vi "Append Image.vi"(0 "PDF Report IN":T24(xcontrol), 1 "Scale (%)":sgl=100.0, 3 "Border":T3={"Show?"=FALSE, "Thickness (point)"=0.5, "Color"=0}, 5 "Image path":path, 9 "Image Ref iTexSharp":refnum<k24>, 11 "error in (no error)":errorcluster, 12 "Caption":string, 14 "Position and indentation":T1={"Alignment"=enum."Center", "X "=0.0, "Y"=0.0, "Indentation"=0.0}) -> (4 "PDF Report OUT":T24(xcontrol), 6 "Image path duplicate":path, 8 "Size (points)":cluster{"TotalHeight":sgl, "TotalWidth":sgl}, 15 "error out":errorcluster)   [LabVIEW 2012]
doc: "The <B>VI</B> appends, to the PDF report, the image from a file. \n\nValid formats: GIF, JPEG, PNG and BMP.\n\n<B>FRANÇAIS</B>\nLe <B>VI</B> ajoute, au rapport PDF, l'image provenant d'un fichier.\n\nFormats valides : GIF, JPEG, PNG et BMP.\n\nVersion 1.0\nDeveloped by Jean-Marc Simard\nCopyright © 2010, Exaprom Inc.\nAll rights reserved.\nLicense: BSD\n\nWith iTextSharp 4.1.6 (http://itextsharp.sourceforge.net)\nunder Mozilla Public License Version 1.1\n(http://www.mozilla.org/MPL/MPL-1.1.html)"
uses:
  C:/Users/MaxCorp/Documents/GitHub/TopView/DLL/itextsharp.dll
  GitHub/TopView/DLL/itextsharp.dll
  Controls/Font size.ctl
  Controls/Font color.ctl
  Controls/Font cluster.ctl
  Controls/Texte alignement.ctl
  Controls/Line spacing.ctl
  Controls/Paragraphe cluster.ctl
  Controls/Image aligment.ctl
  Controls/Image border.ctl
  Controls/PDF Report Xcontrol/PDF Report.xctl
  Controls/Image alignment and position.ctl
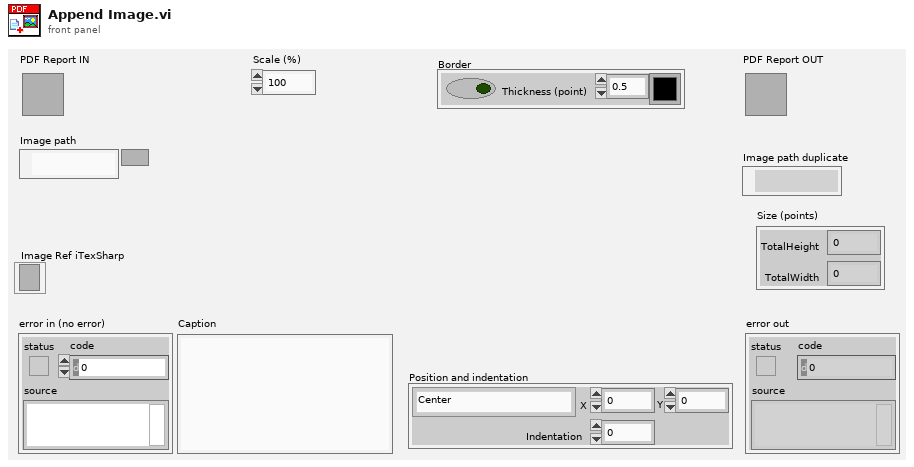
[diagram p1: front panel]
types:
  T1 = typedef "Image alignment and position.ctl" = cluster{"Alignment":T2, "X ":sgl, "Y":sgl, "Indentation":sgl}
  T2 = typedef "Image aligment.ctl" = enum16{"Absolute (X,Y) in mm", "Left", "Center", "Right", "Left (textwrap)", "Right (textwrap)"}
  T3 = typedef "Image border.ctl" = cluster{"Show?":bool, "Thickness (point)":sgl, "Color":u32}
  T4 = typedef "Font cluster.ctl" = cluster{"Name":string, "Size":T5, "Color":T6, "Style":cluster{"Bold":bool, "Italic":bool, "Underline":bool, "Strikeout":bool}}
  T5 = typedef "Font size.ctl" = sgl
  T6 = typedef "Font color.ctl" = u32
  T7 = typedef "Unit.ctl" = enum16{"inch", "mm"}
  T8 = typedef "Paragraphe cluster.ctl" = cluster{" Aligment":T9, "Line spacing":T10}
  T9 = typedef "Texte alignement.ctl" = enum16{"Select", "CENTER", "JUSTIFY", "LEFT", "RIGHT"}
  T10 = typedef "Line spacing.ctl" = enum16{"Select", "1.0", "1.5", "2.0"}
  T11 = typedef "Page dimensions.ctl" = cluster{"Start at page":i32, "Orientation":T12, "widht":sgl, "height":sgl, "Margin left":sgl, "Margin right":sgl, "Margin top":sgl, "Margin bottom":sgl}
  T12 = typedef "Page Orientation.ctl" = enum16{"Portrait", "Landscape"}
  T13 = typedef "Image or Table Caption.ctl" = cluster{"Caption":string, "Separator":string, "Position":enum16{"Above", "Below"}}
  T14 = typedef "Header Footer [ ].ctl" = T15[]
  T15 = typedef "Header Footer cluster.ctl" = cluster{"Start page":i32, "Type":T16, "Alignment":T17, "Vertical Alignement":T18, "Image (%)":sgl, "Page #":T19, "Text":string, "Path":string, "Font":T4, "Font refnum":refnum<k24>, "Line":cluster{"Line":T20, "Thickness (points)":sgl, "Colour":T6}}
  T16 = typedef "Header Footer Type.ctl" = enum16{"Select", "Text", "Text + hyperlink", "Page number", "Image", "Image + hyperlink"}
  T17 = typedef "Header footer horiz alignment.ctl" = enum16{"Left", "Center", "Right"}
  T18 = typedef "Cell Vertical alignment.ctl" = enum16{"TOP", "MIDDLE", "BOTTOM"}
  T19 = typedef "Page number.ctl" = cluster{"Text 1":string, "Text 2":string, "Text 3":string}
  T20 = typedef "Header Footer Line.ctl" = enum16{"No line", "Horizontal line"}
  T21 = typedef "Watermark cluster2.ctl" = cluster{"Show? (F)":bool, "Type":enum16{"Image", "Text"}, "Opacity (%)":sgl, "Rotate(°)":sgl, "Position":cluster{"Position":T22, "X":sgl, "Y":sgl}, "Image path":path, "Scaled(%)":sgl, "Image refnum":refnum<k24>, "Text":string, "Font":cluster{"Name":string, "Size":T5, "Color":T6}, "Font refnum":refnum<k24>, "Alignment":T17, "Automatic":bool}
  T22 = typedef "Watermark Position.ctl" = enum16{"Absolute", "Center (page)", "Center (text section)"}
  T23 = typedef "System Fonts.ctl" = cluster{"Font name [ ]":string[], "Font and file names [ ]":cluster{"Font name":string, "File name":string}[]}
  T24 = cluster{"Document":refnum<k24>, "Writer":refnum<k24>, "Default Font":refnum<k24>, "Default Font cluster":T4, "Path":path, "Unit (default = mm)":T7, "Paragraphe cluster":T8, "Pages dimensions [ ]":T11[], "Captions":cluster{"Image":T13, "Image counter":u16, "Table":T13, "Table counter":u16, "Font":T4}, "Header":T14, "Footer":T14, "Watermark ":T21, "Actual VI name":string, "System Fonts":T23}
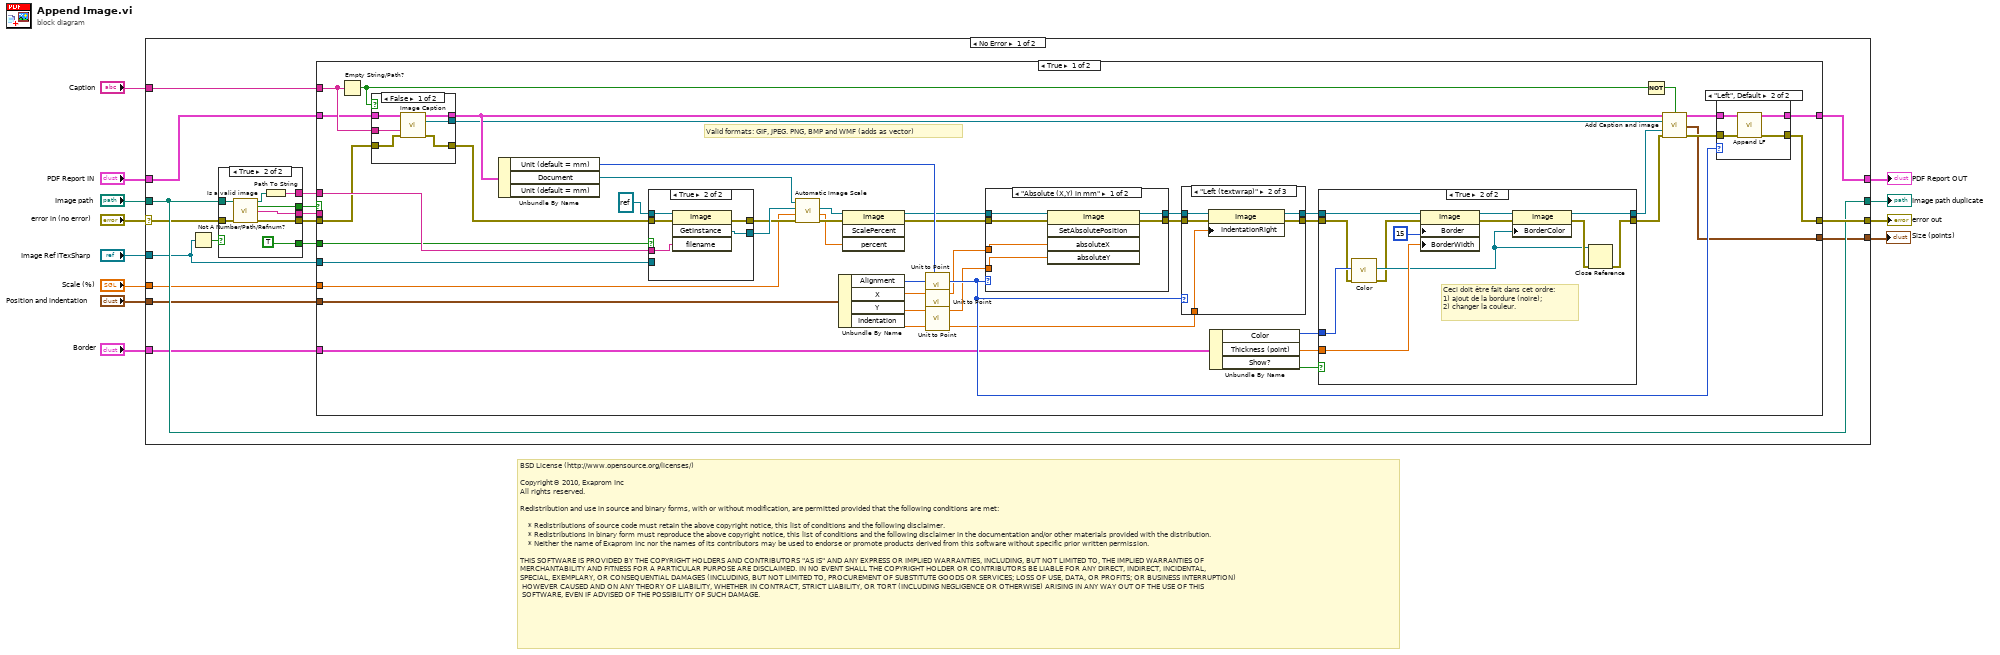
[diagram p0: block diagram]
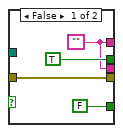
[diagram p2: hidden frame]
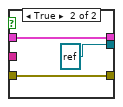
[diagram p5: hidden frame]
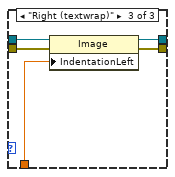
[diagram p7: hidden frame]
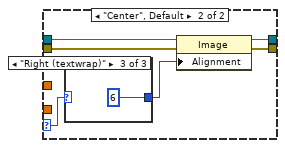
[diagram p9: hidden frame]
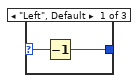
[diagram p10: hidden frame]
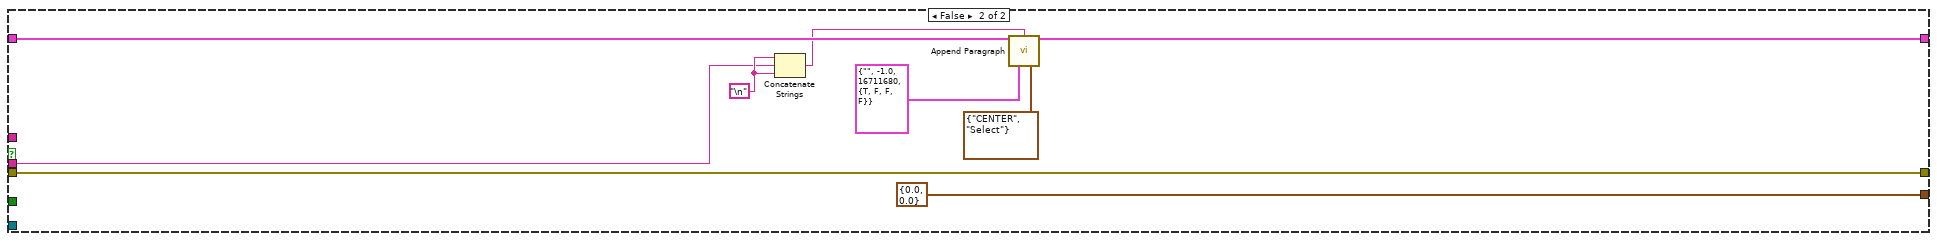
[diagram p12: hidden frame]
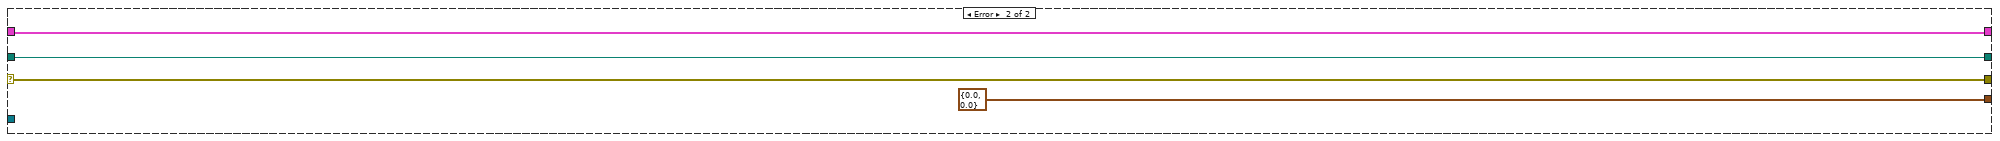
[diagram p13: hidden frame]
diagram:
  # "BSD License (http://www.opensource.org/licenses/)\n\nCopyright© 2010, Exaprom Inc\nAll rights reserved.\n\nRedistribution and use in source and binary forms, with or without modification, are permitted provided that the following conditions are met:\n\n    * Redistributions of source code must retain the above copyright notice, this list of conditions and the following disclaimer.\n    * Redistributions in binary form must reproduce the above copyright notice, this list of conditions and the following disclaimer in the documentation and/or other materials provided with the distribution.\n    * Neither the name of Exaprom Inc nor the names of its contributors may be used to endorse or promote products derived from this software without specific prior written permission.\n\nTHIS SOFTWARE IS PROVIDED BY THE COPYRIGHT HOLDERS AND CONTRIBUTORS \"AS IS\" AND ANY EXPRESS OR IMPLIED WARRANTIES, INCLUDING, BUT NOT LIMITED TO, THE IMPLIED WARRANTIES OF \nMERCHANTABILITY AND FITNESS FOR A PARTICULAR PURPOSE ARE DISCLAIMED. IN NO EVENT SHALL THE COPYRIGHT HOLDER OR CONTRIBUTORS BE LIABLE FOR ANY DIRECT, INDIRECT, INCIDENTAL,\nSPECIAL, EXEMPLARY, OR CONSEQUENTIAL DAMAGES (INCLUDING, BUT NOT LIMITED TO, PROCUREMENT OF SUBSTITUTE GOODS OR SERVICES; LOSS OF USE, DATA, OR PROFITS; OR BUSINESS INTERRUPTION)\n HOWEVER CAUSED AND ON ANY THEORY OF LIABILITY, WHETHER IN CONTRACT, STRICT LIABILITY, OR TORT (INCLUDING NEGLIGENCE OR OTHERWISE) ARISING IN ANY WAY OUT OF THE USE OF THIS\n SOFTWARE, EVEN IF ADVISED OF THE POSSIBILITY OF SUCH DAMAGE."
  n1 = case shown="No Error" "error in (no error)" {
    selector: "error in (no error)" -> [w14 w163]
    tunnel: [w22 w162] -> w7
    tunnel: [w29 w163] -> w12
    tunnel: "PDF Report IN" -> [w24 w162]
    tunnel: "Image path" -> [w25 w161]
    tunnel: [w25 w161] -> w9
    tunnel: "Caption" -> [w23 _]
    tunnel: "Image Ref iTexSharp" -> [w19 _]
    tunnel: "Border" -> [w18 _]
    tunnel: "Position and indentation" -> [w17 _]
    tunnel: "Scale (%)" -> [w16 _]
    tunnel: [w15 cluster{"TotalHeight":sgl, "TotalWidth":sgl} {"TotalHeight"=0.0, "TotalWidth"=0.0}] -> w1
    frame No Error {
      n2 = Not A Number/Path/Refnum?(number/path/refnum=w19) -> (NaN/Path/Refnum?=w21:bool)
      n3 = case shown="True" w21 {
        tunnel: [w31 w40] -> w28
        tunnel: [TRUE ("Valid Image?") w35] -> w27
        tunnel: [w30 w39] -> w26
        tunnel: w25 -> [_ w38]
        tunnel: [FALSE TRUE] -> w20
        tunnel: w14 -> [w30 w36]
        tunnel: [w31 w34] -> w13
        frame False {
          w31 = ""
        }
        frame True {
          n4 = call "Is a valid image.vi"("Image path"=w38, "error in (no error)"=w36) -> ("dup path"=w41:path, "Valid Image?"=w35:bool, "Message"=w34:string, "error out"=w39:errorcluster)  [unwired: 10 out]
          n5 = Path To String(path=w41) -> (string=w40:string)
        }
      }
      n6 = case shown="True" w27 {
        tunnel: [w55 w152] -> w29
        tunnel: w28 -> [w81 _]
        tunnel: w26 -> [w53 w152]
        tunnel: w24 -> [w57 w159]
        tunnel: w23 -> [w68 _]
        tunnel: [w56 w157] -> w22
        tunnel: w20 -> [w67 _]
        tunnel: w19 -> [w66 _]
        tunnel: w18 -> [w65 _]
        tunnel: w17 -> [w63 _]
        tunnel: w16 -> [w43 _]
        tunnel: [w45 cluster{"TotalHeight":sgl, "TotalWidth":sgl} {"TotalHeight"=0.0, "TotalWidth"=0.0}] -> w15
        tunnel: w13 -> [_ w151]
        frame True {
          # "Valid formats: GIF, JPEG. PNG, BMP and WMF (adds as vector)"
          n7 = Empty String/Path?(string/path=w68) -> (empty?=w50:bool)
          n8 = case shown="False" w50 {
            tunnel: [w105 w108] -> w52
            tunnel: w57 -> [w104 w108]
            tunnel: w68 -> [w103 _]
            tunnel: [w102 w107] -> w69
            tunnel: [w101 refnum<k24> refnum ("Paragraph Refnum")] -> w47
            tunnel: w53 -> [w100 w107]
            frame False {
              n9 = call "Image Caption.vi"("PDF Report IN"=w104, "Caption IN"=w103, "error IN"=w100) -> ("PDF Report OUT"=w105:T24, "Paragraph Refnum"=w101:refnum<k24>, "error OUT"=w102:errorcluster)  [unwired: 4 in, 6 out]
            }
            frame True {
              (unwired) sgl 2.0 ("Largeur (default unit)")
              (unwired) u32 0
              (unwired) refnum<k24> refnum ("Cell ref")
              (unwired) sgl 0.0 ("TotalHeight")
            }
          }
          n10 = Unbundle By Name(w52) -> ("Unit (default = mm)"=w85:T7, "Document"=w70:refnum<k24>)  [unwired: 1 out]
          n11 = case shown="True" w67 {
            tunnel: refnum<k24> refnum ("image") -> [_ w99]
            tunnel: w81 -> [_ w98]
            tunnel: [w93 w97] -> w78
            tunnel: [w94 w96] -> w76
            tunnel: w69 -> [w94 w95]
            tunnel: w66 -> [w93 _]
            frame False {
            }
            frame True {
              n12 = invoke class="Image" method="GetInstance"(reference=w99, error in=w95, "filename"=w98) -> (error out=w96:errorcluster, "GetInstance"=w97:refnum<k24>)  [unwired: 1 in, 2 out]
            }
          }
          n13 = call "Automatic Image Scale.vi"("error in (no error)"=w76, "Scale percent IN"=w43, "GetInstanceImage IN"=w78, "Document"=w70) -> ("error out"=w75:errorcluster, "Scale percent OUT"=w74:sgl, "GetInstanceImage OUT"=w77:refnum<k24>)  [unwired: 2 in, 3 out]
          n14 = Unbundle By Name(w63) -> ("Alignment"=w86:T2, "X"=w60:sgl, "Y"=w61:sgl, "Indentation"=w62:sgl)
          n15 = invoke class="Image" method="ScalePercent"(reference=w77, error in=w75, "percent"=w74) -> (reference out=w83:refnum<k24>, error out=w84:errorcluster)  [unwired: 1 in, 2 out]
          n16 = call "Unit to Point.vi"("X unit"=w60, "Unit (default = mm)"=w85) -> ("X point"=w80:sgl)  [unwired: 7 out]
          n17 = call "Unit to Point.vi"("X unit"=w61, "Unit (default = mm)"=w85) -> ("X point"=w79:sgl)  [unwired: 7 out]
          n18 = call "Unit to Point.vi"("X unit"=w62, "Unit (default = mm)"=w85) -> ("X point"=w42:sgl)  [unwired: 7 out]
          n19 = case shown="\"Absolute (X,Y) in mm\"" w86 {
            selector: w86 -> [_ w141]
            tunnel: [w140 w146] -> w72
            tunnel: [w139 w143] -> w71
            tunnel: w84 -> [w138 w144]
            tunnel: w83 -> [w137 w145]
            tunnel: w80 -> [w136 _]
            tunnel: w79 -> [w135 _]
            frame "Absolute (X,Y) in mm" {
              n20 = invoke class="Image" method="SetAbsolutePosition"(reference=w137, error in=w138, "absoluteX"=w136, "absoluteY"=w135) -> (reference out=w140:refnum<k24>, error out=w139:errorcluster)  [unwired: 1 in, 3 out]
            }
            frame "Center", Default {
              n21 = case shown="\"Right (textwrap)\"" w141 {
                selector: w141 -> [w147 w149 _]
                tunnel: [w148 w149 6] -> w142
                frame "Left", Default {
                  n22 = Decrement(x=w147) -> (x-1=w148:T2)
                }
                frame "Left (textwrap)" {
                }
                frame "Right (textwrap)" {
                }
              }
              n23 = property class="Image"(reference=w145, error in=w144, "Alignment"=w142) -> (reference out=w146:refnum<k24>, error out=w143:errorcluster)
            }
          }
          n24 = case shown="\"Left (textwrap)\"" w86 {
            tunnel: [w110 w112 w120] -> w73
            tunnel: w72 -> [w110 w115 w117]
            tunnel: [w109 w113 w119] -> w59
            tunnel: w71 -> [w109 w114 w118]
            tunnel: w42 -> [_ w111 w116]
            frame "Left", Default {
            }
            frame "Left (textwrap)" {
              n25 = property class="Image"(reference=w115, error in=w114, "IndentationRight"=w111) -> (reference out=w112:refnum<k24>, error out=w113:errorcluster)
            }
            frame "Right (textwrap)" {
              n26 = property class="Image"(reference=w117, error in=w118, "IndentationLeft"=w116) -> (reference out=w120:refnum<k24>, error out=w119:errorcluster)
            }
          }
          n27 = Unbundle By Name(w65) -> ("Color"=w54:u32, "Thickness (point)"=w58:sgl, "Show?"=w64:bool)
          n28 = case shown="True" w64 {
            tunnel: w73 -> [w122 w131]
            tunnel: [w122 w132] -> w48
            tunnel: [w121 w129] -> w49
            tunnel: w59 -> [w121 w124]
            tunnel: w54 -> [_ w126]
            tunnel: w58 -> [_ w128]
            frame False {
            }
            frame True {
              # "Ceci doit être fait dans cet ordre:\n1) ajout de la bordure (noire);\n2) changer la couleur."
              n29 = call "Color.vi"("error in (no error)"=w124, "Color"=w126) -> ("error out"=w123:errorcluster, "Color"=w125:refnum<k24>)  [unwired: 8 out]
              n30 = property class="Image"(reference=w131, error in=w123, "Border"=15, "BorderWidth"=w128) -> (reference out=w127:refnum<k24>, error out=w133:errorcluster)
              n31 = property class="Image"(reference=w127, error in=w133, "BorderColor"=w125) -> (reference out=w132:refnum<k24>, error out=w130:errorcluster)
              n32 = Close Reference(reference=w125, error in (no error)=w130) -> (error out=w129:errorcluster)
            }
          }
          n33 = Not(x=w50) -> (.not. x?=w44:bool)
          n34 = call "Add Caption and image.vi"("PDF Report IN"=w52, "Caption?"=w44, "Paragraph Refnum"=w47, "Image Ref iTexSharp"=w48, "error in (no error)"=w49) -> ("PDF Report OUT"=w51:T24, "Size (points)"=w45:cluster{"TotalHeight":sgl, "TotalWidth":sgl}, "error out"=w46:errorcluster)  [unwired: 8 out]
          n35 = case shown="\"Left\", Default" w86 {
            tunnel: w51 -> [w87 w92]
            tunnel: [w87 w91] -> w56
            tunnel: [w88 w90] -> w55
            tunnel: w46 -> [w88 w89]
            frame "Left (textwrap)", "Right (textwrap)" {
            }
            frame "Left", Default {
              n36 = call "Append LF.vi"("PDF Report IN"=w92, "error in (no error)"=w89) -> ("PDF Report duplicate"=w91:T24, "error out"=w90:errorcluster)  [unwired: 1 in, 11 out]
            }
          }
        }
        frame False {
          w156 = "\n"
          n37 = Concatenate Strings(w156, w151, w156) -> (w155:string)
          n38 = call "Append Paragraph.vi"("PDF Report"=w159, "Text"=w155, "Font"=T4 {"Name"="", "Size"=-1.0, "Color"=16711680, "Style"={"Bold"=TRUE, "Italic"=FALSE, "Underline"=FALSE, "Strikeout"=FALSE}}, "Paragraph properties"=T8 {" Aligment"=enum."CENTER", "Line spacing"=enum."Select"}) -> ("PDF Report duplicate"=w157:T24)  [unwired: 3 in, 8 out]
        }
      }
    }
    frame Error {
    }
  }
  "error out" <- w12
  "PDF Report OUT" <- w7
  "Image path duplicate" <- w9
  "Size (points)" <- w1
